vi "Remove From Tree.vi"(8 "error in (no error)":errorcluster, 11 "NodeRef In":refnum<data-value>) -> (0 "error out":errorcluster, 1 "Children":refnum<data-value>[](array[refnum]), 2 "Parent":refnum<data-value>, 3 "NodeRef":refnum<data-value>)   [LabVIEW 2020, in "PicoG-ParserLexer.lvlib" / "Node.lvclass"]
uses:
  Node.lvclass
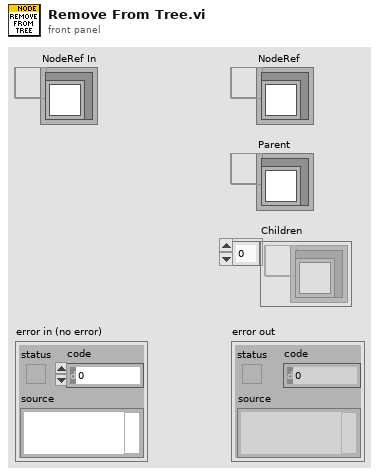
[diagram p1: front panel]
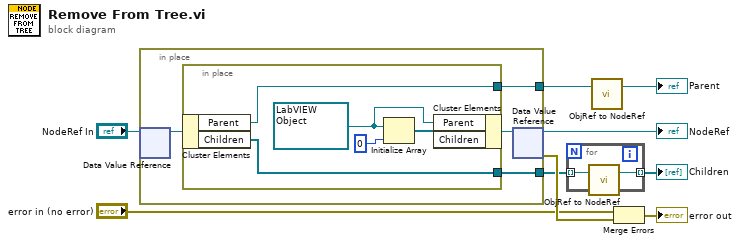
[diagram p0: block diagram]
diagram:
  n1 = in-place {
    in-place-border: [w12] -> w6
    in-place-border: [w10] -> w2
    n2 = in-place-dvr #1("NodeRef In") -> (w13:refnum<class "Node.lvclass">)  [unwired: 1 out]
    n3 = in-place {
      in-place-border: [w18] -> w12
      in-place-border: [w15] -> w10
      w14 = refnum<data-value> refnum ("Sibling")
      n4 = in-place-cluster #2(w13) -> ("Parent"=w15:refnum<data-value>, "Children"=w18:refnum<data-value>[])
      n5 = Initialize Array(w14, 0 ("dimension size")) -> (w17:refnum<data-value>[])
      n6 = in-place-cluster #2("Parent"=w14, "Children"=w17) -> (w11:refnum<class "Node.lvclass">)
    }
    n7 = in-place-dvr #1(w11) -> (→"NodeRef":refnum<data-value>, w9:errorcluster)
  }
  n8 = for {
    tunnel: w6 -> [w20] mode=indexing
    tunnel: [w19] -> w5 mode=indexing
    n9 = call "ObjRef to NodeRef.vi"("ObjectRef"=w20) -> ("NodeRef"=w19:refnum<data-value>)  [unwired: 2 in]
  }
  "Children" <- w5
  n10 = call "ObjRef to NodeRef.vi"("ObjectRef"=w2) -> ("NodeRef"=→"Parent":refnum<data-value>)  [unwired: 2 in]
  n11 = Merge Errors("error in (no error)", w9) -> (→"error out":errorcluster)
